vi "XYZ Stage-Response validator.vi"(11 "response string":string="AA\r1234\r300") -> (1 "Filtered response":string, 3 "Value":i32)   [LabVIEW 2020]
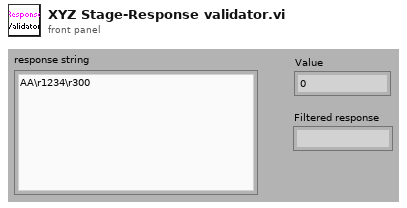
[diagram p1: front panel]
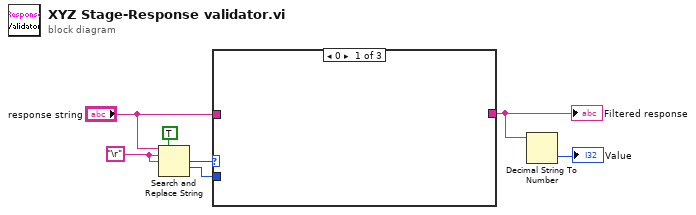
[diagram p0: block diagram]
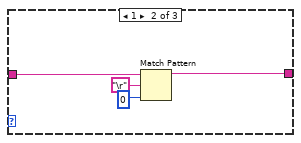
[diagram p2: hidden frame]
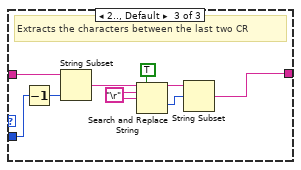
[diagram p3: hidden frame]
diagram:
  w6 = "\r"
  n1 = Search and Replace String(replace all?=TRUE ("replace all? (F)"), input string="response string", search string=w6, replace string=w6) -> (number of replacements=w5:i32, offset past replacement=w4:i32)  [unwired: 4 in, 2 out]
  n2 = case shown="0" w5 {
    tunnel: "response string" -> [_ w10 w20]
    tunnel: w4 -> [_ _ w19]
    tunnel: [_ w8 w12] -> w2
    frame 0 {
    }
    frame 1 {
      n3 = Match Pattern(string=w10, regular expression="\r", offset (0)=0) -> (before substring=w8:string)  [unwired: 3 out]
    }
    frame 2.., Default {
      w15 = "\r"
      # "Extracts the characters between the last two CR"
      n4 = Decrement(x=w19) -> (x-1=w17:i32)
      n5 = String Subset(string=w20, length (rest)=w17) -> (substring=w18:string)  [unwired: 1 in]
      n6 = Search and Replace String(replace all?=TRUE ("replace all? (F)"), input string=w18, search string=w15, replace string=w15) -> (result string=w14:string, offset past replacement=w13:i32)  [unwired: 4 in, 2 out]
      n7 = String Subset(string=w14, offset (0)=w13) -> (substring=w12:string)  [unwired: 1 in]
    }
  }
  "Filtered response" <- w2
  n8 = Decimal String To Number(string=w2) -> (number=→"Value":i32)  [unwired: 2 in, 1 out]
